vi "ExportErrorLog.vi"(8 "error in (no error)":errorcluster, 11 "CDependencyInspection in":refnum<class "CDependencyInspection.lvclass">) -> (0 "error out":errorcluster, 2 "Succeeded?":bool, 3 "CDependencyInspection out":refnum<class "CDependencyInspection.lvclass">)   [LabVIEW 2020, in "DependencyInspection.lvlib" / "CDependencyInspection.lvclass"]
uses:
  CDependencyInspection.lvclass
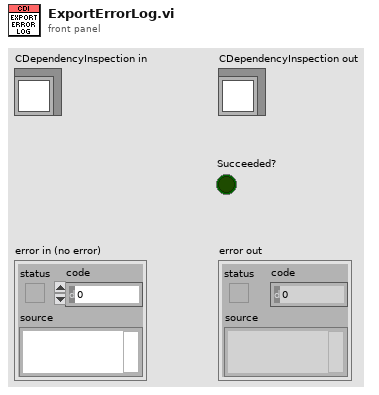
[diagram p1: front panel]
types:
  T1 = enum16{"open", "replace", "create", "open or create", "replace or create", "replace or create with confirmation"}
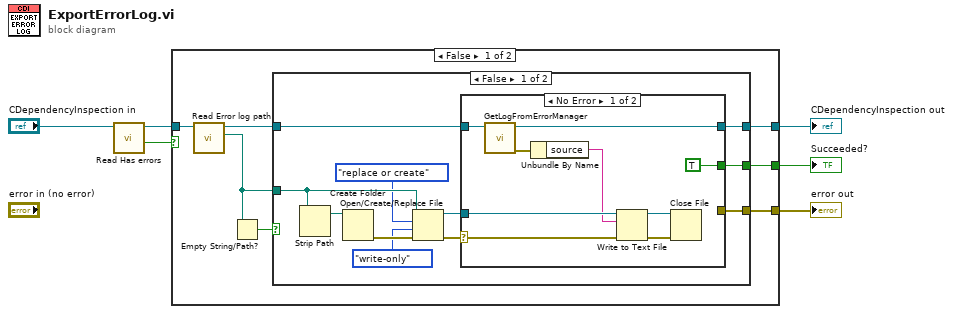
[diagram p0: block diagram]
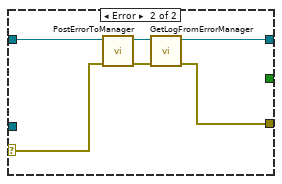
[diagram p2: hidden frame]
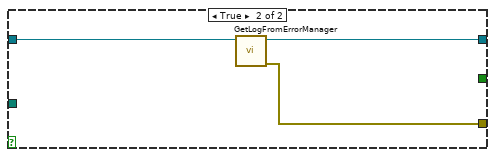
[diagram p3: hidden frame]
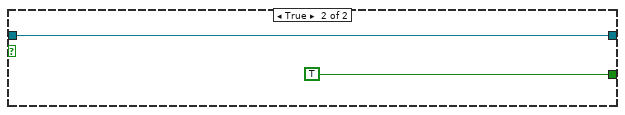
[diagram p4: hidden frame]
diagram:
  n1 = call-dynamic "Read Has errors.vi"("CDependencyInspection in"="CDependencyInspection in") -> ("empty?"=w1:bool, "CDependencyInspection out"=w2:refnum<class "CDependencyInspection.lvclass">)  [unwired: 9 in]
  n2 = case shown="False" w1 {
    tunnel: w2 -> [w11 w44]
    tunnel: [w7 w44] -> w6
    tunnel: [w10 TRUE ("Exit LV?")] -> w5
    tunnel: [w9 _] -> w4
    frame False {
      n3 = call-dynamic "Read Error log path.vi"("CDependencyInspection in"=w11) -> ("Error log path"=w12:path, "CDependencyInspection out"=w8:refnum<class "CDependencyInspection.lvclass">)  [unwired: 9 in]
      n4 = Empty String/Path?(string/path=w12) -> (empty?=w13:bool)
      n5 = case shown="False" w13 {
        tunnel: w12 -> [w22 _]
        tunnel: [w17 w40] -> w9
        tunnel: [w16 _] -> w10
        tunnel: w8 -> [w15 w41]
        tunnel: [w14 w42] -> w7
        frame False {
          n6 = Strip Path(path=w22) -> (stripped path=w24:path)  [unwired: 1 out]
          n7 = Create Folder(path (use dialog)=w24) -> (error out=w23:errorcluster)  [unwired: 2 in, 2 out]
          n8 = Open/Create/Replace File(file path (use dialog)=w22, error in=w23, operation (0:open)=T1."replace or create", access (0:read/write)=enum16{"read/write", "read-only", "write-only"}."write-only") -> (refnum out=w18:refnum<file>, error out=w19:errorcluster)  [unwired: 2 in, 1 out]
          n9 = case shown="No Error" w19 {
            selector: w19 -> [w32 w34]
            tunnel: w18 -> [w33 _]
            tunnel: [_ w36] -> w17
            tunnel: [TRUE ("Exit LV?") _] -> w16
            tunnel: w15 -> [w28 w39]
            tunnel: [w27 w37] -> w14
            frame No Error {
              n10 = call-dynamic "GetLogFromErrorManager.vi"("CDependencyInspection in"=w28) -> ("error out"=w26:errorcluster, "CDependencyInspection out"=w27:refnum<class "CDependencyInspection.lvclass">)  [unwired: 8 in, 1 out]
              n11 = Unbundle By Name(w26) -> ("source"=w25:string)
              n12 = Write to Text File(file (use dialog)=w33, text=w25, error in=w32) -> (refnum out=w31:refnum<file>, error out=w30:errorcluster)  [unwired: 1 in, 1 out]
              n13 = Close File(refnum=w31, error in=w30) -> ()  [unwired: 2 out]
            }
            frame Error {
              n14 = call-dynamic "PostErrorToManager.vi"("error in (no error)"=w34, "CDependencyInspection in"=w39) -> ("error out"=w35:errorcluster, "CDependencyInspection out"=w38:refnum<class "CDependencyInspection.lvclass">)  [unwired: 8 in]
              n15 = call-dynamic "GetLogFromErrorManager.vi"("error in (no error)"=w35, "CDependencyInspection in"=w38) -> ("error out"=w36:errorcluster, "CDependencyInspection out"=w37:refnum<class "CDependencyInspection.lvclass">)  [unwired: 7 in, 1 out]
            }
          }
        }
        frame True {
          n16 = call-dynamic "GetLogFromErrorManager.vi"("CDependencyInspection in"=w41) -> ("error out"=w40:errorcluster, "CDependencyInspection out"=w42:refnum<class "CDependencyInspection.lvclass">)  [unwired: 8 in, 1 out]
        }
      }
    }
    frame True {
    }
  }
  "error out" <- w4
  "CDependencyInspection out" <- w6
  "Succeeded?" <- w5
